vi "Activate_IPS_high_precission_mode.vi"(1 "High Precission":bool, 3 "Address":T1={"Com Port"=1, "ISOBUS Address"=1, "GPIB Address"=24, "Communication"=enum."ISOBUS"}) -> (0 "Address(thru)":T1={"Com Port"=1, "ISOBUS Address"=1, "GPIB Address"=24, "Communication"=enum."ISOBUS"})   [LabVIEW 2019]
uses:
  Oxford Software/Oxsoft/BUSGEN.LLB/OxfordAddress.ctl
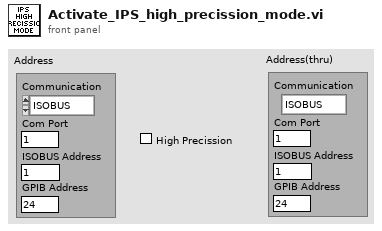
[diagram p1: front panel]
types:
  T1 = typedef "OxfordAddress.ctl" = cluster{"Com Port":i32, "ISOBUS Address":i32, "GPIB Address":i16, "Communication":enum16{"RS232", "ISOBUS", "GPIB", "Gateway"}}
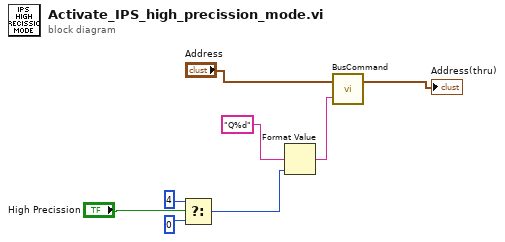
[diagram p0: block diagram]
diagram:
  n1 = Select(t=4, s="High Precission", f=0) -> (s? t:f=w1:i32)
  n2 = Format Value(format string="Q%d", value (0)=w1) -> (output string=w2:string)  [unwired: 1 in]
  n3 = call "BusCommand.vi"("Command"=w2, "Instrument address (in)"="Address") -> ("Instrument address (out)"=→"Address(thru)":T1)  [unwired: 1 out]
